vi "lockin_Vsg_multichannel.vi"(9 "B rate":dbl=20060.440145, 10 "Comments":string="test magnet sweep \n\n\n100uV ac + -250 uV dc, time constant 0.5 s\nf=13.46Hz", 11 "ITX folder":string="test - lockinsweepVsg") -> ()   [LabVIEW 2013]
uses:
  <userlib>/LevyLab/PPMS VI/SubVI/ITX_Global.vi
  B field global.vi
  P:/users1/Joe/Lockin-4461_3.0 4461-4462 Multichannel Folder/DAQ-Lockin-SubVI/Lock-in Globles Multiple Inputs and Outputs.vi
  Q:/inst/Leiden measurements VIs/IV measurement/Sub VIs/Global Value.vi
panel:
  in  "Tab Control":enum32{"Control", "Data"}(tab)
  in  "OSC Configuration 2":T1(array[cluster])=[[{"Signal Type"=enum."Sine Wave", "DC"=0.0, "Amplitude"=0.0, "frequency"=13.46, "Phase"=0.0}, {"Signal Type"=enum."Sine Wave", "DC"=0.0, "Amplitude"=0.0005, "frequency"=13.46, "Phase"=0.0}], [{"Signal Type"=enum."Sine Wave", "DC"=0.0, "Amplitude"=0.0, "frequency"=13.46, "Phase"=0.0}, {"Signal Type"=enum."Sine Wave", "DC"=0.0, "Amplitude"=0.0, "frequency"=13.46, "Phase"=0.0}], [{"Signal Type"=enum."Sine Wave", "DC"=0.0, "Amplitude"=0.0, "frequency"=13.46, "Phase"=0.0}, {"Signal Type"=enum."Sine Wave", "DC"=0.0, "Amplitude"=0.0, "frequency"=13.46, "Phase"=0.0}], [{"Signal Type"=enum."Sine Wave", "DC"=0.0, "Amplitude"=0.0, "frequency"=13.46, "Phase"=0.0}, {"Signal Type"=enum."Sine Wave", "DC"=0.0, "Amplitude"=0.0, "frequency"=13.46, "Phase"=0.0}]] {"frequency" step=0.001 format="%.3p"; "Amplitude" format="%0.2p"; "DC" min=-0.99 max=0.99 format="%.2p"}
  in  "Vo":dbl=-0.06 format="%#_3p"
  in  "Vmax":dbl=0.06 format="%#_3p"
  in  "Vmin":dbl=0.06 format="%#_3p"
  in  "dV":dbl=0.0001 format="%#_3p"
  out "KH Status":string
  out "T (mK)":dbl=20060.440145
  in  "wait between Vsgs":u32
  in  "Initial wait":u32=5000
  out "Bx, By, Bz (T)":dbl[](array[numeric])=[1.0606601717798214, 1.0606601717798212, 9.184850993605148e-17]
  in  "# of lockins":i32=6
  in  "Card":i32=3
  in  "Output":i32
  out "Lockins":cluster{"Y":dbl[], "Y":dbl[]}[](graph)
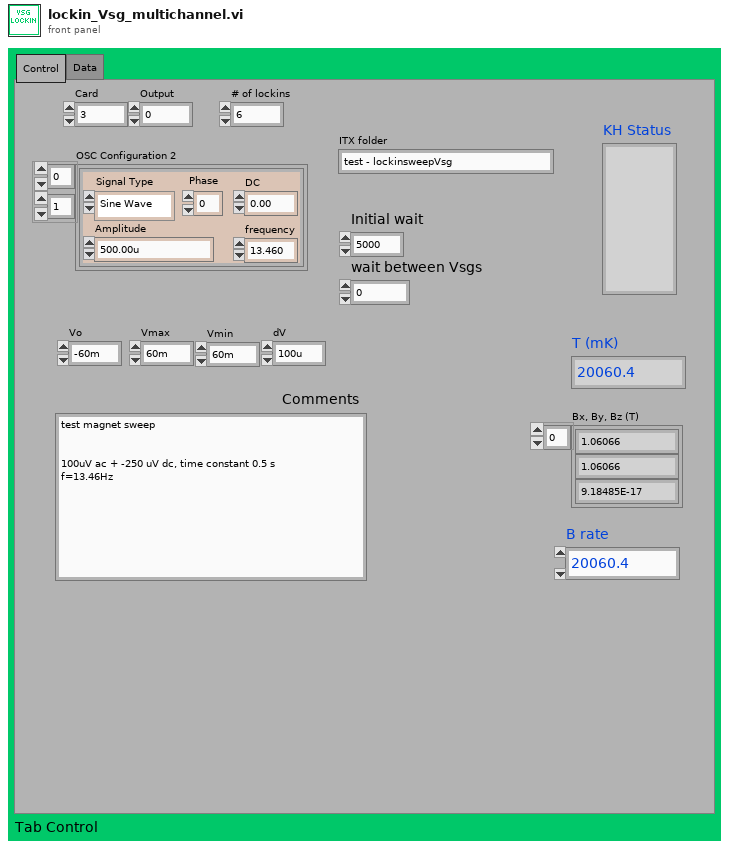
[diagram p1: front panel]
types:
  T1 = cluster{"Signal Type":enum16{"Sine Wave", "Triangle Wave", "Square Wave", "Sawtooth Wave"}, "DC":dbl, "Amplitude":dbl, "frequency":dbl, "Phase":dbl}[][]
  T2 = cluster{"Signal Type":enum16{"Sine Wave", "Triangle Wave", "Square Wave", "Sawtooth Wave"}, "DC":dbl, "Amplitude":dbl, "frequency":dbl, "Phase":dbl}
  T3 = cluster{"Channel":u16, "Gain":u16, "Shunt Resistor":u16, "Measure":u16}[]
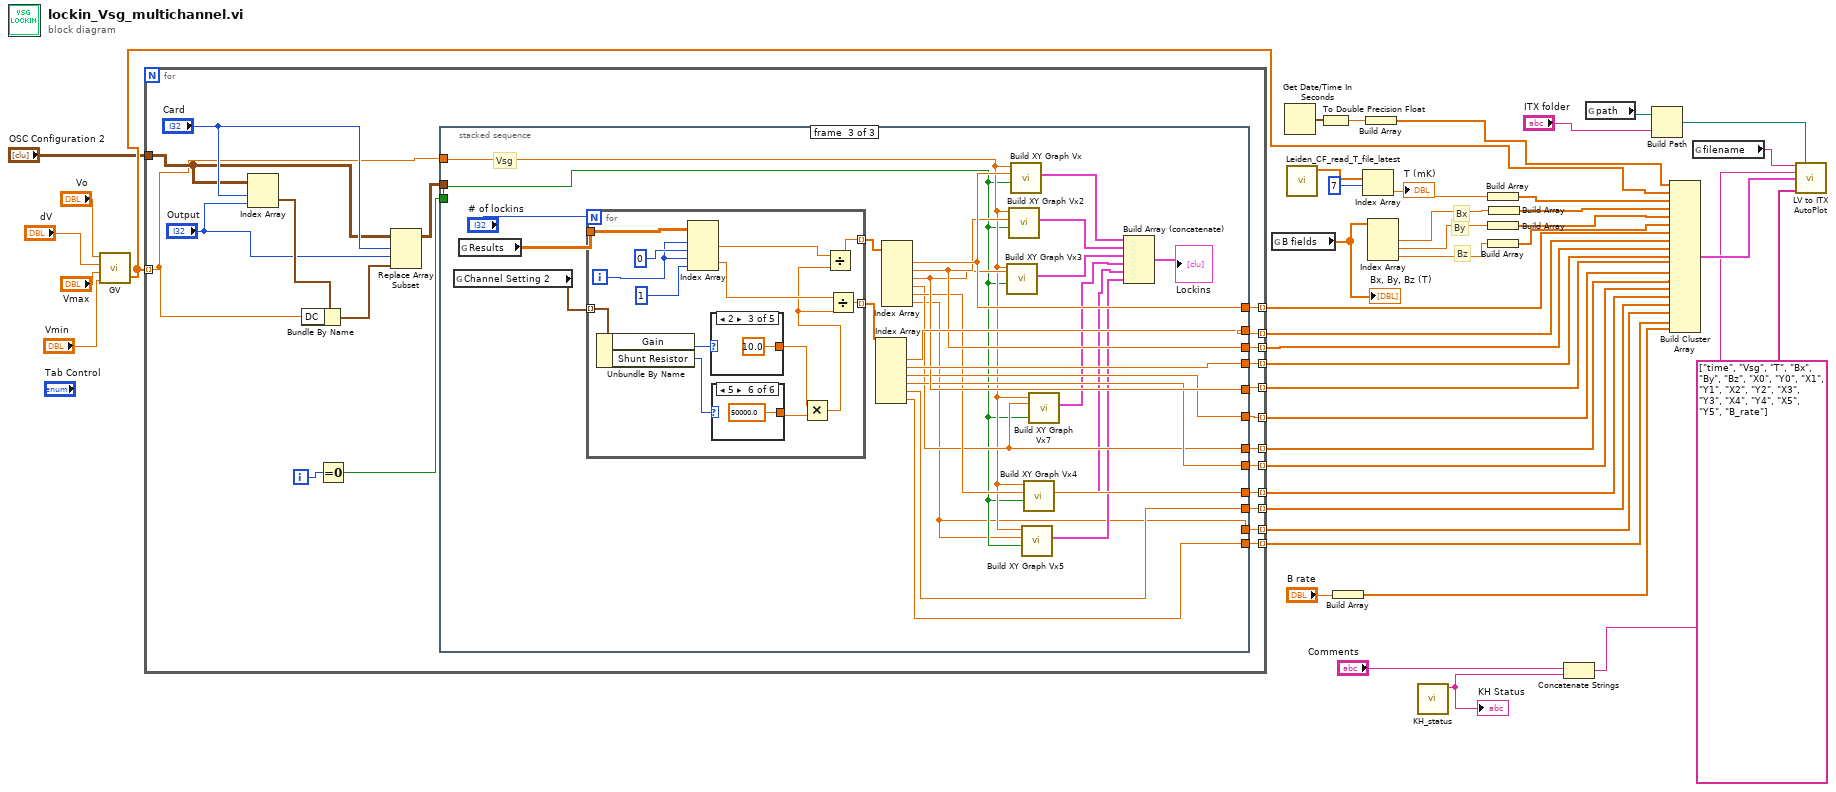
[diagram p0: block diagram]
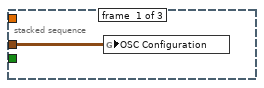
[diagram p2: hidden frame]
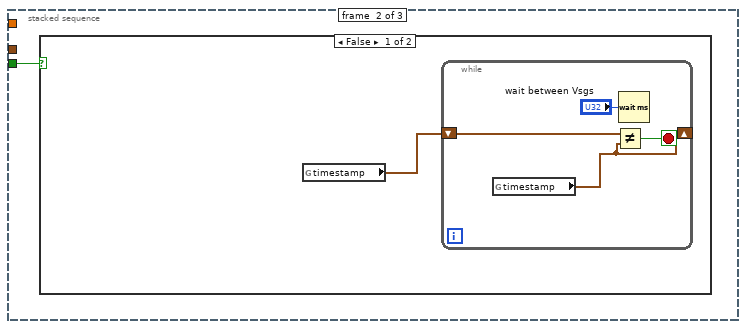
[diagram p3: hidden frame]
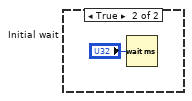
[diagram p4: hidden frame]
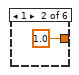
[diagram p6: hidden frame]
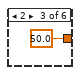
[diagram p7: hidden frame]
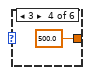
[diagram p8: hidden frame]
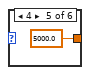
[diagram p9: hidden frame]
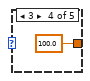
[diagram p12: hidden frame]
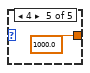
[diagram p13: hidden frame]
diagram:
  # "Bz"
  # "By"
  # "Bx"
  n1 = call <userlib>:"GV.vi"("Vmin"="Vmin", "Vmax"="Vmax", "dV"="dV", "Vo"="Vo") -> ("Waveform Graph"=w10:dbl[])  [unwired: 1 in]
  n2 = for {
    tunnel: "OSC Configuration 2" -> [w63]
    tunnel: w10 -> [w53] mode=indexing
    tunnel: [w59] -> w25 mode=indexing
    tunnel: [w58] -> w27 mode=indexing
    tunnel: [w57] -> w26 mode=indexing
    tunnel: [w56] -> w24 mode=indexing
    tunnel: [w55] -> w14 mode=indexing
    tunnel: [w54] -> w13 mode=indexing
    tunnel: [w52] -> w12 mode=indexing
    tunnel: [w51] -> w11 mode=indexing
    tunnel: [w50] -> w7 mode=indexing
    tunnel: [w49] -> w6 mode=indexing
    tunnel: [w48] -> w5 mode=indexing
    tunnel: [w44] -> w1 mode=indexing
    i -> [w61]
    n3 = Index Array(array=w63, index (row)="Card", index (col)="Output") -> (element=w47:T2)
    n4 = Bundle By Name(cluster=w47, "DC"=w53) -> (w46:T2)
    n5 = Equal To 0?(x=w61) -> (x = 0?=w60:bool)
    n6 = Replace Array Subset(array=w63, new element=w46, index (row)="Card", index (col)="Output") -> (w62:T1)
    n7 = stacked-sequence {
      tunnel: w62 -> [w65 _ _]
      tunnel: w53 -> [_ _ w78]
      tunnel: w60 -> [_ w66 w77]
      tunnel: [_ _ w87] -> w59
      tunnel: [_ _ w89] -> w58
      tunnel: [_ _ w88] -> w57
      tunnel: [_ _ w86] -> w56
      tunnel: [_ _ w85] -> w55
      tunnel: [_ _ w84] -> w54
      tunnel: [_ _ w79] -> w52
      tunnel: [_ _ w83] -> w51
      tunnel: [_ _ w82] -> w50
      tunnel: [_ _ w81] -> w49
      tunnel: [_ _ w80] -> w48
      tunnel: [_ _ w73] -> w44
      frame #0 {
        n8 = global write "Lock-in Globles Multiple Inputs and Outputs.vi" "OSC Configuration"(w65) -> ()
      }
      frame #1 {
        n9 = case shown="False" w66 {
          frame False {
            n10 = global read "Lock-in Globles Multiple Inputs and Outputs.vi" "timestamp"() -> (w67:timestamp)
            n11 = while {
              shift-right: [w68] -> _
              shift-left: w67 -> [w71]
              stop <- w70 stop-if-true
              n12 = global read "Lock-in Globles Multiple Inputs and Outputs.vi" "timestamp"() -> (w68:timestamp)
              n13 = Not Equal?(x=w71, y=w68) -> (x != y?=w70:bool)
              n14 = Wait (ms)(milliseconds to wait="wait between Vsgs") -> ()  [unwired: 1 out]
            }
          }
          frame True {
            n15 = Wait (ms)(milliseconds to wait="Initial wait") -> ()  [unwired: 1 out]
          }
        }
      }
      frame #2 {
        # "Vsg"
        n16 = global read "Global Value.vi" "Channel Setting 2"() -> (w92:T3)
        n17 = global read "Lock-in Globles Multiple Inputs and Outputs.vi" "Results"() -> (w94:dbl[][])
        n18 = for {
          N: "# of lockins" -> [_]
          tunnel: w94 -> [w110]
          tunnel: [w103] -> w91 mode=indexing
          tunnel: [w100] -> w90 mode=indexing
          tunnel: w92 -> [w108] mode=indexing
          i -> [w99]
          n19 = Unbundle By Name(w108) -> ("Gain"=w109:u16, "Shunt Resistor"=w107:u16)
          n20 = Index Array(array=w110, index (row) #1=w99, index (col) #1=0 ("disabled index (col)"), index (row) #2=w99, index (col) #2=1 ("disabled index (col)")) -> (element #1=w104:dbl, element #2=w102:dbl)
          n21 = case shown="2" w109 {
            selector: w109 -> [w119 w120 _ _ _]
            tunnel: [w119 w120 10.0 100.0 1000.0] -> w106
            frame 0, Default {
            }
            frame 1 {
            }
            frame 2 {
            }
            frame 3 {
            }
            frame 4 {
            }
          }
          n22 = case shown="5" w107 {
            selector: w107 -> [w113 _ _ _ _ _]
            tunnel: [w113 1.0 50.0 500.0 5000.0 50000.0] -> w105
            frame 0, Default {
            }
            frame 1 {
            }
            frame 2 {
            }
            frame 3 {
            }
            frame 4 {
            }
            frame 5 {
            }
          }
          n23 = Multiply(x=w106, y=w105) -> (x*y=w101:dbl)
          n24 = Divide(x=w104, y=w101) -> (x/y=w103:dbl)
          n25 = Divide(x=w102, y=w101) -> (x/y=w100:dbl)
        }
        n26 = Index Array(array=w90) -> (element #1=w88:dbl, element #2=w86:dbl, element #3=w84:dbl, element #4=w83:dbl, element #5=w81:dbl, element #6=w80:dbl)  [unwired: 6 in]
        n27 = Index Array(array=w91) -> (element #1=w89:dbl, element #2=w87:dbl, element #3=w85:dbl, element #4=w79:dbl, element #5=w82:dbl, element #6=w73:dbl)  [unwired: 6 in]
        n28 = call "Build XY Graph Vx3"("Reset"=w77, "Y Input"=w85, "X Input"=w78) -> ("XY Graph"=w96:cluster{"Y":dbl[], "Y":dbl[]}[])  [unwired: 2 in, 6 out]
        n29 = call "Build XY Graph Vx2"("Reset"=w77, "Y Input"=w87, "X Input"=w78) -> ("XY Graph"=w97:cluster{"Y":dbl[], "Y":dbl[]}[])  [unwired: 2 in, 6 out]
        n30 = call "Build XY Graph Vx"("Reset"=w77, "Y Input"=w89, "X Input"=w78) -> ("XY Graph"=w98:cluster{"Y":dbl[], "Y":dbl[]}[])  [unwired: 2 in, 6 out]
        n31 = call "Build XY Graph Vx5"("Reset"=w77, "Y Input"=w73, "X Input"=w78) -> ("XY Graph"=w74:cluster{"Y":dbl[], "Y":dbl[]}[])  [unwired: 2 in, 6 out]
        n32 = call "Build XY Graph Vx4"("Reset"=w77, "Y Input"=w82, "X Input"=w78) -> ("XY Graph"=w75:cluster{"Y":dbl[], "Y":dbl[]}[])  [unwired: 2 in, 6 out]
        n33 = call "Build XY Graph Vx7"("Reset"=w77, "Y Input"=w79, "X Input"=w78) -> ("XY Graph"=w76:cluster{"Y":dbl[], "Y":dbl[]}[])  [unwired: 2 in, 6 out]
        n34 = Build Array (concatenate)(w98, w97, w96, w76, w75, w74) -> (→"Lockins":cluster{"Y":dbl[], "Y":dbl[]}[])
      }
    }
  }
  n35 = global read "B field global.vi" "B fields"() -> (w9:dbl[])
  "Bx, By, Bz (T)" <- w9
  n36 = Get Date/Time In Seconds() -> (seconds since 1Jan1904=w17:timestamp)
  n37 = call "Leiden_CF_read_T_file_latest.vi"() -> ("T array"=w20:dbl[])  [unwired: 11 in]
  n38 = To Double Precision Float(number=w17) -> (double precision float=w16:dbl)
  n39 = Build Array("B rate") -> (w2:dbl[])
  n40 = Index Array(array=w20, index=7) -> (element=w32:dbl)
  "T (mK)" <- w32
  n41 = Build Array(w16) -> (w15:dbl[])
  n42 = Index Array(array=w9) -> (element #1=w23:dbl, element #2=w22:dbl, element #3=w21:dbl)  [unwired: 3 in]
  n43 = call "KH_status.vi"() -> ("KH Status"=w8:string)  [unwired: 11 in]
  "KH Status" <- w8
  n44 = Build Array(w32) -> (w31:dbl[])
  n45 = Build Array(w22) -> (w29:dbl[])
  n46 = Build Array(w21) -> (w28:dbl[])
  n47 = Build Array(w23) -> (w30:dbl[])
  n48 = Concatenate Strings("Comments", w8) -> (w18:string)
  n49 = global read "ITX_Global.vi" "path"() -> (w38:path)
  n50 = Build Path(base path=w38, name or relative path="ITX folder") -> (appended path=w37:path)
  n51 = Build Cluster Array(w15, w10, w31, w30, w29, w28, w27, w26, w25, w24, w14, w13, w12, w11, w7, w6, w1, w5, w2) -> (w35:cluster{"Waveform Graph":dbl[]}[])
  n52 = global read "ITX_Global.vi" "filename"() -> (w36:string)
  n53 = call <userlib>:"LV to ITX AutoPlot.vi"("filename"=w36, "path"=w37, "Notes"=w18, "Data"=w35, "wavenames (.Vx, etc)"=string[] ["time", "Vsg", "T", "Bx", "By", "Bz", "X0", "Y0", "X1", "Y1", "X2", "Y2", "X3", "Y3", "X4", "Y4", "X5", "Y5", "B_rate"]) -> ()  [unwired: 10 in, 1 out]
